vi "Test Read Bit.vi"() -> ()   [LabVIEW 2014]
uses:
  ALPHA5 RS485/typedefs/Port Selection Info.ctl
  ALPHA5 RS485/ALPHA5 RS485.lvlib
panel:
  in  "Specified Num in":u8=1
  out "FC":u8
  out "bits array":bool[](array[boolean])
  out "byte num":u8
  out "error out":errorcluster
  out "CRC Match":bool
  in  "Address":u16=65535 format="%.0x"
  in  "error in (no error)":errorcluster caption="error in（no error）"
  in  "Port Selection Info In":T1={"Port Name"="", "Amplifier Num"=1, "Baud Rate"=38400, "Char Formation"=enum."0"} {"Baud Rate" items=["38400"=38400, "19200"=19200, "9600"=9600, "115200"=0]; "Amplifier Num" max=31}
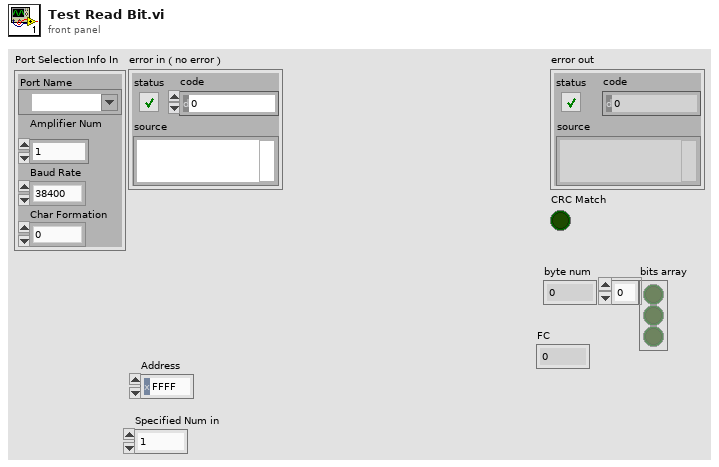
[diagram p1: front panel]
types:
  T1 = typedef "ALPHA5 RS485.lvlib/Port Selection Info.ctl" = cluster{"Port Name":refnum<visa-resource-name>, "Amplifier Num":u8, "Baud Rate":u32, "Char Formation":enum16{"0", "1", "2", "3", "4", "5"}}
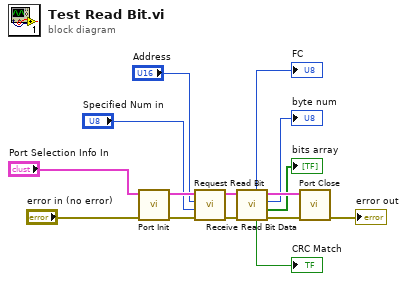
[diagram p0: block diagram]
diagram:
  n1 = call "Port Init.vi"("error in (no error)"="error in (no error)", "Port Selection Info In"="Port Selection Info In") -> ("error out"=w7:errorcluster, "Port Selection Info Out"=w8:T1)  [unwired: 8 in]
  n2 = call "Request Read Bit.vi"("error in (no error)"=w7, "Specified Num in"="Specified Num in", "Address"="Address", "Port Selection Info"=w8) -> ("error out"=w14:errorcluster, "Port Selection Info Out"=w15:T1)  [unwired: 5 in, 1 out]
  n3 = call "Receive Read Bit Data.vi"("error in (no error)"=w14, "Port Selection Info"=w15) -> ("error out"=w10:errorcluster, "bits array"=→"bits array":bool[], "byte num"=→"byte num":u8, "Port Selection Info Out"=w11:T1, "CRC Match"=→"CRC Match":bool, "FC"=→"FC":u8)  [unwired: 3 in, 1 out]
  n4 = call "Port Close.vi"("error in (no error)"=w10, "Port Selection Info In"=w11) -> ("error out"=→"error out":errorcluster)  [unwired: 9 in]
